vi "getWaveForm.vi"(0 "tiempo (s)":sgl, 1 "#samples":u32, 2 "Amplitud":dbl, 3 "frecuencia":dbl, 4 "Fs (S/s)":dbl, 5 "df":dbl[](array[numeric])) -> (7 "Waveform":waveform(dbl)(graph))   [LabVIEW 2010]
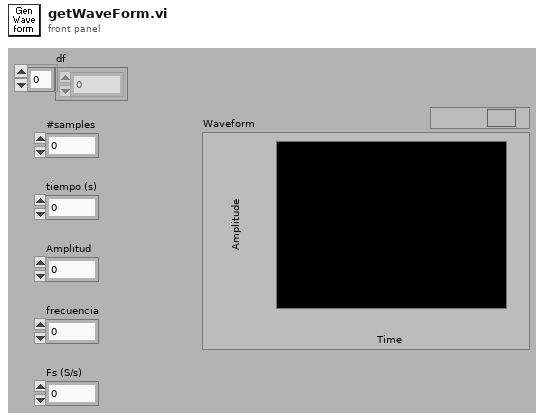
[diagram p1: front panel]
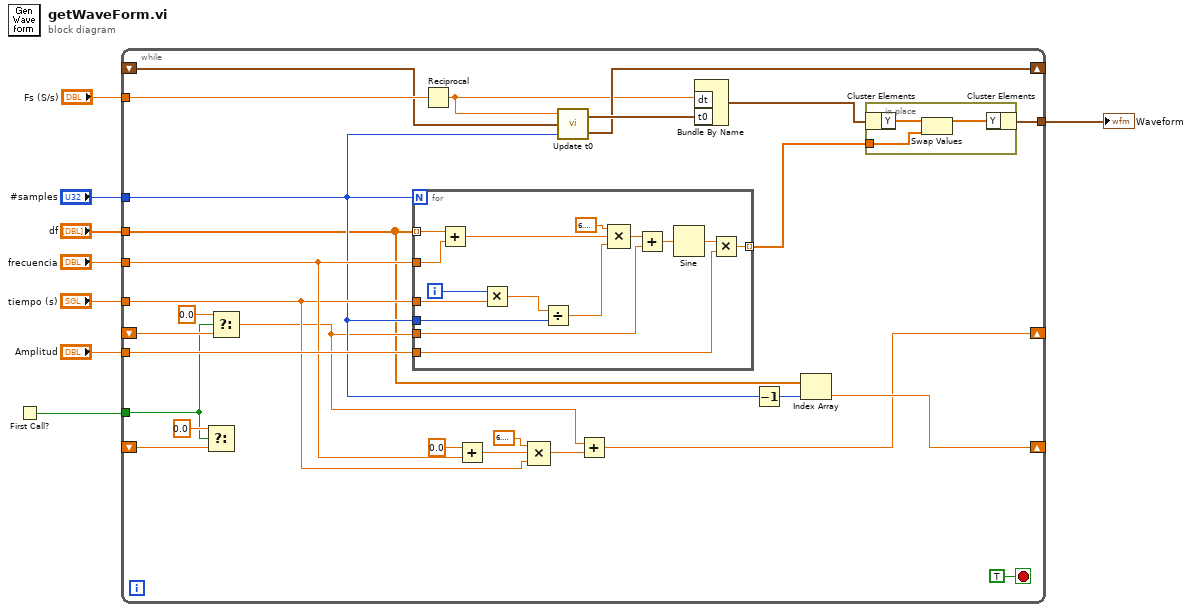
[diagram p0: block diagram]
diagram:
  n1 = First Call?() -> (First Call?: T/F=w1:bool)
  n2 = while {
    tunnel: "#samples" -> [w20]
    tunnel: "tiempo (s)" -> [w23]
    tunnel: "frecuencia" -> [w26]
    tunnel: "Amplitud" -> [w34]
    shift-right: [w21] -> _
    shift-left: _ -> [w17]
    tunnel: "Fs (S/s)" -> [w33]
    shift-right: [w29] -> _
    shift-left: _ -> [w31]
    tunnel: [w18] -> w8
    tunnel: "df" -> [w10]
    shift-right: [w27] -> _
    shift-left: _ -> [w13]
    tunnel: w1 -> [w12]
    stop <- TRUE stop-if-true
    n3 = Select(t=0.0, s=w12, f=w13) -> ()  [unwired: 1 out]
    n4 = Select(t=0.0, s=w12, f=w17) -> (s? t:f=w16:dbl)
    n5 = for {
      N: w20 -> [_]
      tunnel: w23 -> [w52]
      tunnel: w26 -> [w43]
      tunnel: w16 -> [w49]
      tunnel: w34 -> [w47]
      tunnel: w20 -> [w41]
      tunnel: w10 -> [w40] mode=indexing
      tunnel: [w39] -> w9 mode=indexing
      i -> [w53]
      n6 = Add(x=w40, y=w43) -> (x+y=w42:dbl)
      n7 = Multiply(x=w53, y=w52) -> (x*y=w51:sgl)
      n8 = Divide(x=w51, y=w41) -> (x/y=w45:sgl)
      n9 = Compound Arithmetic op=MULTIPLY(6.283185307179586, w42, w45) -> (w44:dbl)
      n10 = Add(x=w44, y=w49) -> (x+y=w50:dbl)
      n11 = Sine(x=w50) -> (sin(x)=w48:dbl)
      n12 = Multiply(x=w48, y=w47) -> (x*y=w39:dbl)
    }
    n13 = Reciprocal(x=w33) -> (1/x=w19:dbl)
    n14 = Add(x=0.0, y=w26) -> (x+y=w24:dbl)
    n15 = Compound Arithmetic op=MULTIPLY(6.283185307179586, w24, w23) -> (w22:dbl)
    n16 = call "Update t0.vi"("#samples"=w20, "t0 IN"=w31, "dt"=w19) -> ("tf new"=w29:timestamp, "t0 OUT"=w30:timestamp)
    n17 = Add(x=w16, y=w22) -> (x+y=w21:dbl)
    n18 = Bundle By Name("dt"=w19, "t0"=w30) -> (w32:waveform(dbl))  [unwired: 1 in]
    n19 = Decrement(x=w20) -> (x-1=w28:u32)
    n20 = Index Array(array=w10, index=w28) -> (element=w27:dbl)
    n21 = in-place {
      in-place-border: w9 -> [w36]
      n22 = in-place-cluster #1(w32) -> ("Y"=w38:dbl[])
      n23 = Swap Values(12:w38, 14:w36) -> (1:w37:dbl[])  [unwired: 1 in, 1 out]
      n24 = in-place-cluster #1("Y"=w37) -> (w18:waveform(dbl))
    }
  }
  "Waveform" <- w8
